vi "LM_II_27_07_16.vi"   [LabVIEW 2015]
uses:
  <vilib>/NXT/Block Support/NXT_OutputPort.ctl
  <vilib>/NXT/Block Support/NXT_InputPort.ctl
  <vilib>/NXT/Block Support/NXT_MessageMailbox.ctl
  <vilib>/NXT/Subs/MotorOutput.ctl
  <vilib>/NXT/Block Support/NXT_TimerIndex.ctl
  <vilib>/NXT/Dual Mode Library/Sound/Tone.vi
  <vilib>/NXT/Dual Mode Library/Waits/Wait_Num.vi
  <vilib>/NXT/Dual Mode Library/Sensors/Touch_Pressed.vi
  <vilib>/NXT/NXTIO Xnodes/NXTIONodeSubVIs/NXTMoveMotors.vi
  <vilib>/NXT/NXTIO Xnodes/NXTIONodeSubVIs/NXTStopMotors.vi
  <vilib>/NXT/Dual Mode Library/Motors/ResetMotor.vi
  <vilib>/NXT/Dual Mode Library/Motors/Rotation.vi
  <vilib>/NXT/Dual Mode Library/Sensors/Reset_Timer.vi
  <vilib>/NXT/Dual Mode Library/Sensors/Read_Timer.vi
  <vilib>/NXT/Subs/LVHSConnector.ctl
  <vilib>/NXT/NXTIO Xnodes/AddressXNode/NXTIOAddress.xnode
  <vilib>/NXT/NXTIO Xnodes/NXTIOXNode/NXTIO.xnode
  <vilib>/NXT/LegoClasses/BrickReference/BrickReference.lvclass
types:
  T1 = typedef "LVHSConnector.ctl" = refnum<class "BrickReference.lvclass">
  T2 = typedef "NXT_MessageMailbox.ctl" = u8
  T3 = typedef "NXT_InputPort.ctl" = u32
  T4 = typedef "NXT_OutputPort.ctl" = u8
  T5 = cluster{"Port":T4, "Port":T4, "Port":T4, "Port":T4}
  T6 = cluster{"Output Port":T4, "Output Port 2":T4, "Output Port 3":T4, "Output Port 4":T4}
  T7 = typedef "MotorOutput.ctl" = u8
  T8 = typedef "NXT_TimerIndex.ctl" = u8
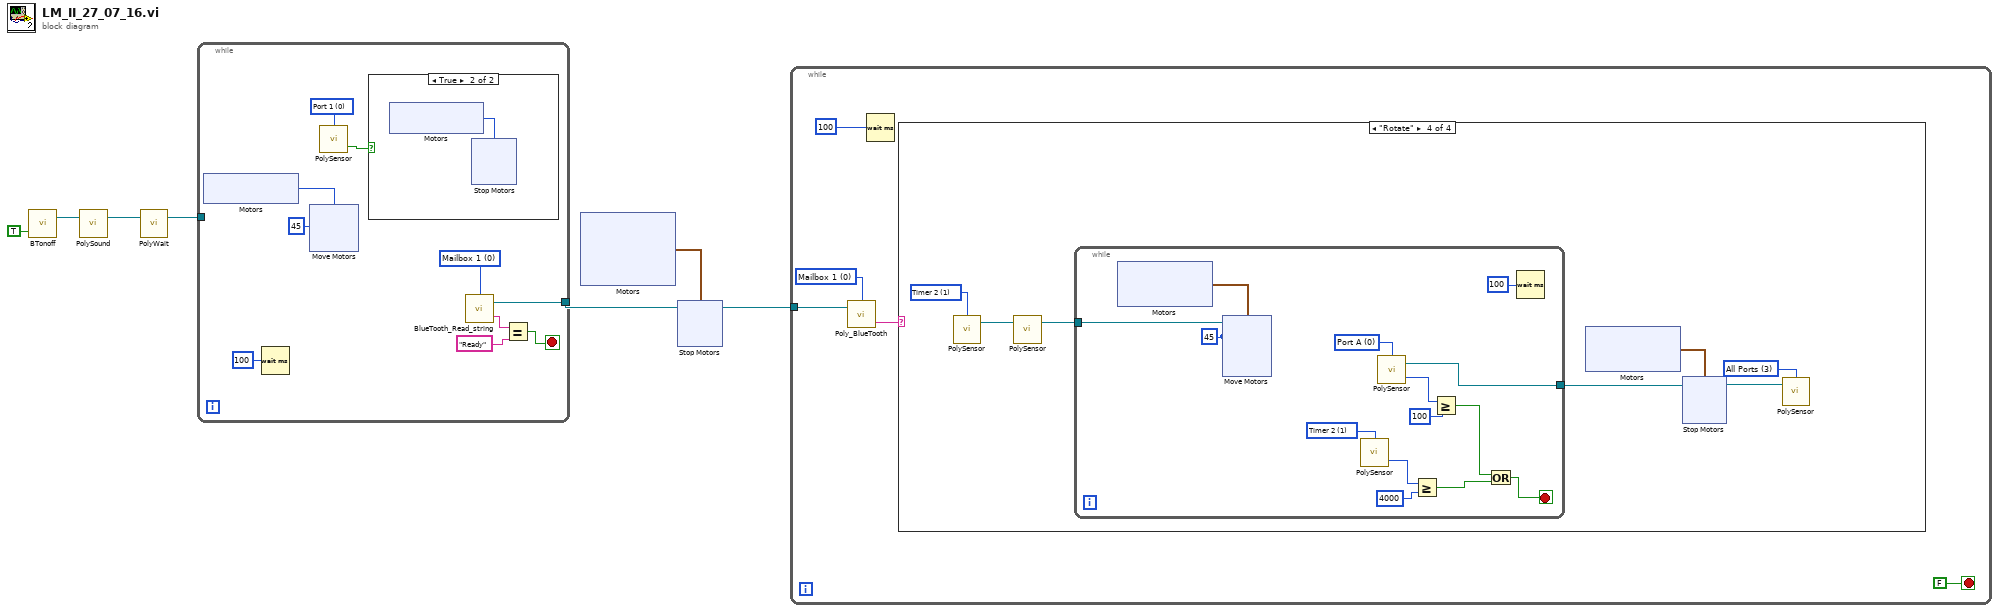
[diagram p0: block diagram]
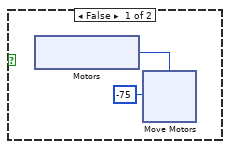
[diagram p2: hidden frame]
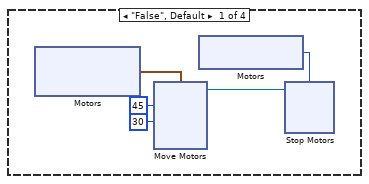
[diagram p3: hidden frame]
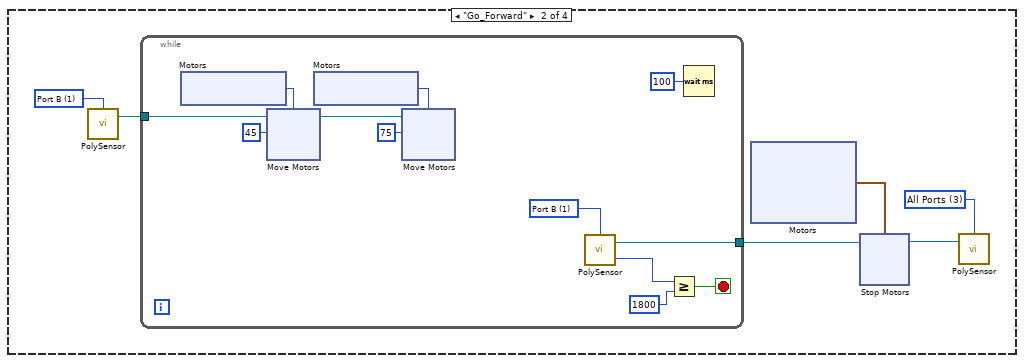
[diagram p4: hidden frame]
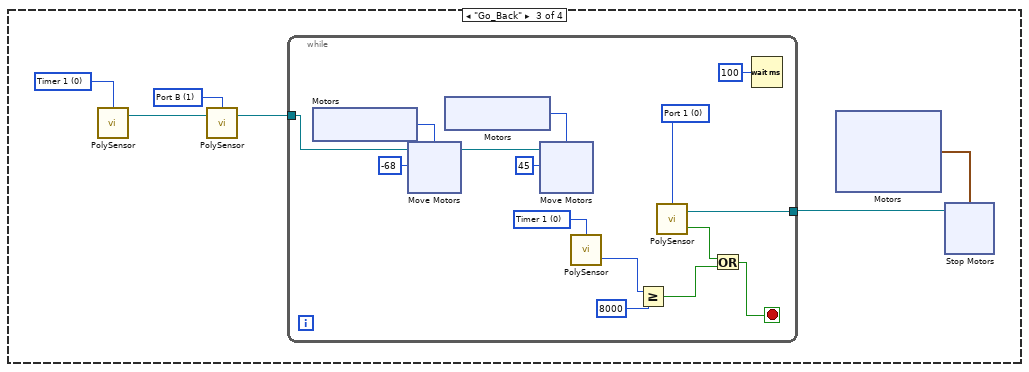
[diagram p5: hidden frame]
diagram:
  n1 = call <vilib>:"BTonoff.vi"("On/Off"=TRUE) -> ("NXT/EV3"=w2:T1)  [unwired: 2 in, 1 out]
  n2 = call-poly <vilib>:"PolySound.vi"("NXT/EV3"=w2) -> ("NXT/EV3"=w4:T1)  [unwired: 3 in]
  n3 = call-poly <vilib>:"PolyWait.vi"("NXT/EV3"=w4) -> ("NXT/EV3"=w1:T1)  [unwired: 3 in]
  n4 = while {
    tunnel: [w9] -> w6
    tunnel: w1 -> [_]
    stop <- w13 stop-if-true
    w10 = T2 0 items=["Mailbox 1", "Mailbox 2", "Mailbox 3", "Mailbox 4", "Mailbox 5", "Mailbox 6", "Mailbox 7", "Mailbox 8", "Mailbox 9", "Mailbox 10"] ("Mailbox")
    w16 = T3 0 items=["Port 1", "Port 2", "Port 3", "Port 4"] ("Port (Port 1)")
    n5 = xnode "Motors"() -> ("Motor"=w11:T4)
    n6 = Wait (ms)(milliseconds to wait=u32 100) -> ()  [unwired: 1 out]
    n7 = xnode "Move Motors"("Power/Speed 1"=i8 45, "Motors"=w11) -> ()  [unwired: 1 in, 1 out]
    n8 = call-poly <vilib>:"PolySensor.vi"("Port (Port 1)"=w16) -> ("Yes / No"=w15:bool)  [unwired: 2 in, 1 out]
    n9 = case shown="True" w15 {
      frame False {
        n10 = xnode "Motors"() -> ("Motor"=w26:T4)
        n11 = xnode "Move Motors"("Power/Speed 1"=i8 -75, "Motors"=w26) -> ()  [unwired: 1 in, 1 out]
      }
      frame True {
        n12 = xnode "Motors"() -> ("Motor"=w36:T4)
        n13 = xnode "Stop Motors"("Motors"=w36) -> ()  [unwired: 1 in, 1 out]
      }
    }
    n14 = call <vilib>:"BlueTooth_Read_string.vi"("Mailbox"=w10) -> ("Message"=w8:string, "NXT/EV3"=w9:T1)  [unwired: 2 in]
    n15 = Equal?(x=w8, y="Ready") -> (x = y?=w13:bool)
  }
  n16 = xnode "Motors"() -> ("Motor"=w7:T5)
  n17 = xnode "Stop Motors"("Motors"=w7, "NXT/EV3"=w6) -> ("NXT/EV3"=w5:T1)
  n18 = while {
    tunnel: w5 -> [w44]
    stop <- FALSE stop-if-true
    w45 = T2 0 items=["Mailbox 1", "Mailbox 2", "Mailbox 3", "Mailbox 4", "Mailbox 5", "Mailbox 6", "Mailbox 7", "Mailbox 8", "Mailbox 9", "Mailbox 10"] ("Mailbox")
    n19 = call-poly <vilib>:"Poly_BlueTooth.vi"("NXT/EV3"=w44, "Mailbox"=w45) -> ("Message"=w43:string)  [unwired: 1 in, 1 out]
    n20 = Wait (ms)(milliseconds to wait=u32 100) -> ()  [unwired: 1 out]
    n21 = case shown="\"Rotate\"" w43 {
      frame "False", Default {
        n22 = xnode "Motors"() -> ("Motor"=w51:cluster{"Port":T4, "Port":T4})
        n23 = xnode "Move Motors"("Power/Speed 2"=i8 30, "Power/Speed 1"=i8 45, "Motors"=w51) -> ("NXT/EV3"=w49:T1)  [unwired: 1 in]
        n24 = xnode "Motors"() -> ("Motor"=w52:T4)
        n25 = xnode "Stop Motors"("Motors"=w52, "NXT/EV3"=w49) -> ()  [unwired: 1 out]
      }
      frame "Go_Forward" {
        w71 = T7 3 items=["Port A"=0, "Port B"=1, "Port C"=2, "Ports A & B"=4, "Ports A & C"=5, "Ports B & C"=6, "All Ports"=3] ("Port (All Ports)")
        w73 = T7 1 items=["Port A"=0, "Port B"=1, "Port C"=2, "Ports A & B"=4, "Ports A & C"=5, "Ports B & C"=6, "All Ports"=3] ("Port (All Ports)")
        n26 = call-poly <vilib>:"PolySensor.vi"("Port (All Ports)"=w73) -> ("NXT/EV3"=w72:T1)  [unwired: 3 in]
        n27 = while {
          tunnel: w72 -> [w83]
          tunnel: [w81] -> w69
          stop <- w91 stop-if-true
          w84 = T4 1 items=["Port A", "Port B", "Port C", "Port D"] ("Port (Port A)")
          n28 = xnode "Motors"() -> ("Motor"=w87:T4)
          n29 = xnode "Move Motors"("Power/Speed 1"=i8 45, "Motors"=w87, "NXT/EV3"=w83) -> ("NXT/EV3"=w82:T1)
          n30 = xnode "Motors"() -> ("Motor"=w85:T4)
          n31 = xnode "Move Motors"("Power/Speed 1"=i8 75, "Motors"=w85, "NXT/EV3"=w82) -> ()  [unwired: 1 out]
          n32 = call-poly <vilib>:"PolySensor.vi"("Port (Port A)"=w84) -> ("Angle of Rotation"=w80:i32, "NXT/EV3"=w81:T1)  [unwired: 2 in]
          n33 = Greater Or Equal?(x=w80, y=1800) -> (x >= y?=w91:bool)
          n34 = Wait (ms)(milliseconds to wait=u32 100) -> ()  [unwired: 1 out]
        }
        n35 = xnode "Motors"() -> ("Motor"=w70:T5)
        n36 = xnode "Stop Motors"("Motors"=w70, "NXT/EV3"=w69) -> ("NXT/EV3"=w68:T1)
        n37 = call-poly <vilib>:"PolySensor.vi"("NXT/EV3"=w68, "Port (All Ports)"=w71) -> ()  [unwired: 2 in, 1 out]
      }
      frame "Go_Back" {
        w109 = T8 0 items=["Timer 1", "Timer 2", "Timer 3"] ("Timer (Timer 1)")
        w111 = T7 1 items=["Port A"=0, "Port B"=1, "Port C"=2, "Ports A & B"=4, "Ports A & C"=5, "Ports B & C"=6, "All Ports"=3] ("Port (All Ports)")
        n38 = call-poly <vilib>:"PolySensor.vi"("Timer (Timer 1)"=w109) -> ("NXT/EV3"=w108:T1)  [unwired: 3 in]
        n39 = call-poly <vilib>:"PolySensor.vi"("NXT/EV3"=w108, "Port (All Ports)"=w111) -> ("NXT/EV3"=w110:T1)  [unwired: 2 in]
        n40 = while {
          tunnel: [w121] -> w112
          tunnel: w110 -> [w125]
          stop <- w133 stop-if-true
          w122 = T3 0 items=["Port 1", "Port 2", "Port 3", "Port 4"] ("Port (Port 1)")
          w124 = T8 0 items=["Timer 1", "Timer 2", "Timer 3"] ("Timer (Timer 1)")
          n41 = xnode "Motors"() -> ("Motor"=w129:T4)
          n42 = xnode "Move Motors"("Power/Speed 1"=i8 -68, "Motors"=w129, "NXT/EV3"=w125) -> ("NXT/EV3"=w126:T1)
          n43 = xnode "Motors"() -> ("Motor"=w127:T4)
          n44 = xnode "Move Motors"("Power/Speed 1"=i8 45, "Motors"=w127, "NXT/EV3"=w126) -> ()  [unwired: 1 out]
          n45 = call-poly <vilib>:"PolySensor.vi"("Timer (Timer 1)"=w124) -> ("Value (msec)"=w123:u32)  [unwired: 2 in, 1 out]
          n46 = Greater Or Equal?(x=w123, y=u32 8000) -> (x >= y?=w131:bool)
          n47 = call-poly <vilib>:"PolySensor.vi"("Port (Port 1)"=w122) -> ("Yes / No"=w120:bool, "NXT/EV3"=w121:T1)  [unwired: 2 in]
          n48 = Or(x=w120, y=w131) -> (x .or. y?=w133:bool)
          n49 = Wait (ms)(milliseconds to wait=u32 100) -> ()  [unwired: 1 out]
        }
        n50 = xnode "Motors"() -> ("Motor"=w113:T5)
        n51 = xnode "Stop Motors"("Motors"=w113, "NXT/EV3"=w112) -> ()  [unwired: 1 out]
      }
      frame "Rotate" {
        w153 = T8 1 items=["Timer 1", "Timer 2", "Timer 3"] ("Timer (Timer 1)")
        w156 = T7 3 items=["Port A"=0, "Port B"=1, "Port C"=2, "Ports A & B"=4, "Ports A & C"=5, "Ports B & C"=6, "All Ports"=3] ("Port (All Ports)")
        n52 = call-poly <vilib>:"PolySensor.vi"("Timer (Timer 1)"=w153) -> ("NXT/EV3"=w152:T1)  [unwired: 3 in]
        n53 = call-poly <vilib>:"PolySensor.vi"("NXT/EV3"=w152) -> ("NXT/EV3"=w151:T1)  [unwired: 3 in]
        n54 = while {
          tunnel: w151 -> [w166]
          tunnel: [w169] -> w154
          stop <- w174 stop-if-true
          w165 = T8 1 items=["Timer 1", "Timer 2", "Timer 3"] ("Timer (Timer 1)")
          w167 = i8 45 ("Power/Speed 1")
          w171 = T4 0 items=["Port A", "Port B", "Port C", "Port D"] ("Port (Port A)")
          n55 = xnode "Motors"() -> ("Motor"=w168:cluster{"Port":T4, "Port":T4})
          n56 = xnode "Move Motors"("Power/Speed 2"=w167, "Power/Speed 1"=w167, "Motors"=w168, "NXT/EV3"=w166) -> ()  [unwired: 1 out]
          n57 = call-poly <vilib>:"PolySensor.vi"("Timer (Timer 1)"=w165) -> ("Value (msec)"=w164:u32)  [unwired: 2 in, 1 out]
          n58 = call-poly <vilib>:"PolySensor.vi"("Port (Port A)"=w171) -> ("Angle of Rotation"=w170:i32, "NXT/EV3"=w169:T1)  [unwired: 2 in]
          n59 = Greater Or Equal?(x=w164, y=u32 4000) -> (x >= y?=w172:bool)
          n60 = Greater Or Equal?(x=w170, y=100) -> (x >= y?=w173:bool)
          n61 = Or(x=w173, y=w172) -> (x .or. y?=w174:bool)
          n62 = Wait (ms)(milliseconds to wait=u32 100) -> ()  [unwired: 1 out]
        }
        n63 = xnode "Motors"() -> ("Motor"=w157:cluster{"Port":T4, "Port":T4})
        n64 = xnode "Stop Motors"("Motors"=w157, "NXT/EV3"=w154) -> ("NXT/EV3"=w155:T1)
        n65 = call-poly <vilib>:"PolySensor.vi"("NXT/EV3"=w155, "Port (All Ports)"=w156) -> ()  [unwired: 2 in, 1 out]
      }
    }
  }
